vi "Get top coincs to check and grafts.vi"(11 "Coincidences":T1[](array[typedef])) -> (0 "Coincidences to check":T1[](array[typedef]), 1 "Found safe graft spot?":bool, 2 "Coincidences to graft":T1[](array[typedef]))   [LabVIEW 2016]
uses:
  Typedefs/Coincidence.ctl
  Global Variables/Global Resolution.vi
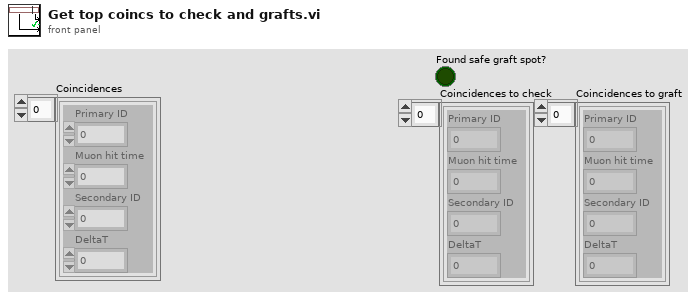
[diagram p1: front panel]
types:
  T1 = typedef "Coincidence.ctl" = cluster{"Primary ID":i8, "Muon hit time":u64, "Secondary ID":i8, "DeltaT":i32}
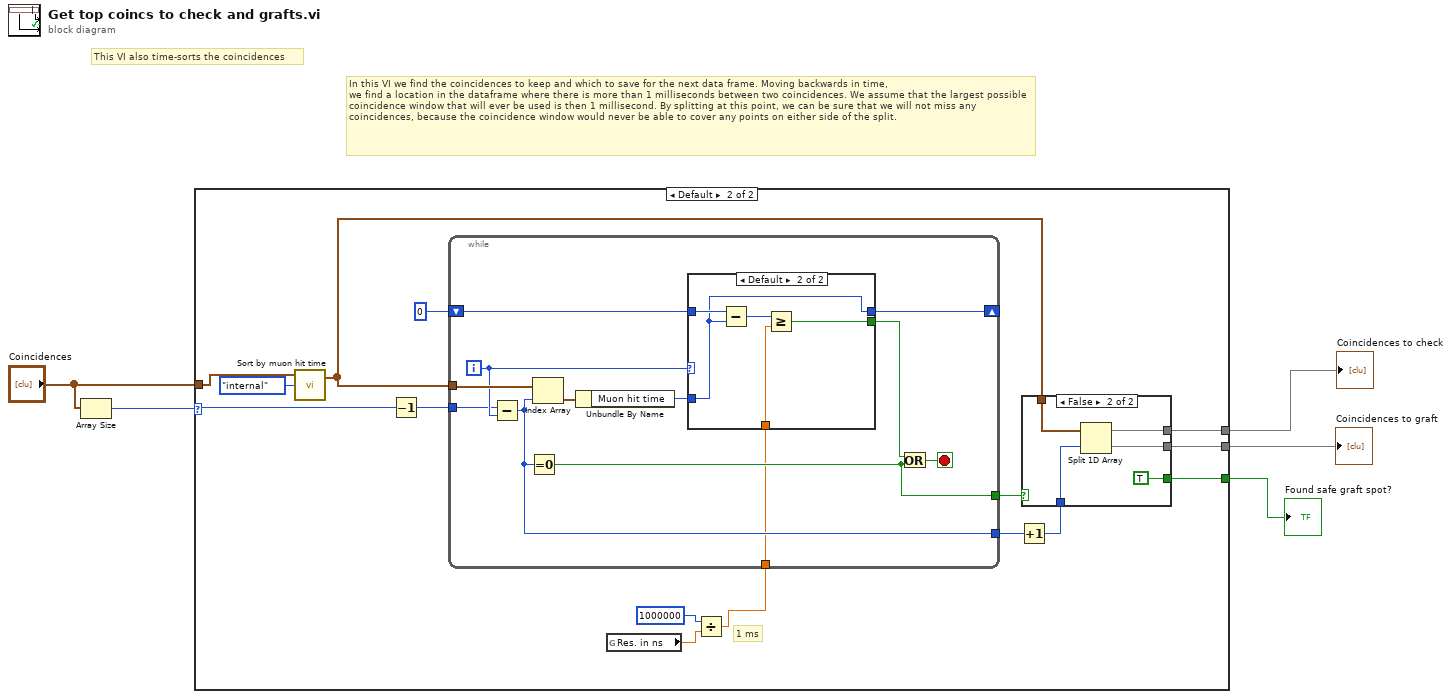
[diagram p0: block diagram]
diagram:
  # "This VI also time-sorts the coincidences"
  # "In this VI we find the coincidences to keep and which to save for the next data frame. Moving backwards in time,\nwe find a location in the dataframe where there is more than 1 milliseconds between two coincidences. We assume that the largest possible coincidence window that will ever be used is then 1 millisecond. By splitting at this point, we can be sure that we will not miss any coincidences, because the coincidence window would never be able to cover any points on either side of the split."
  n1 = Array Size(array="Coincidences") -> (size(s)=w2:i32)
  n2 = case shown="Default" w2 {
    selector: w2 -> [_ w14]
    tunnel: [_ w18] -> w5
    tunnel: [_ w17] -> w4
    tunnel: "Coincidences" -> [_ w8]
    tunnel: [_ w9] -> w1
    frame 0 {
    }
    frame Default {
      # "1 ms"
      n3 = call "Sort by muon hit time.vi"("Type"=enum16{"internal", "saving"}."internal", "Top Coincs internal"=w8) -> ("Coincidences internal"=w6:T1[])  [unwired: 1 in, 1 out]
      n4 = Decrement(x=w14) -> (x-1=w15:i32)
      n5 = global read "Global Resolution.vi" "Res. in ns"() -> (w11:ext)
      n6 = Divide(x=i64 1000000 ("y"), y=w11) -> (x/y=w10:ext)
      n7 = while {
        tunnel: w6 -> [w38]
        tunnel: [w36] -> w19
        shift-right: [w33] -> _
        shift-left: i64 0 ("Muon hit time") -> [w32]
        tunnel: w15 -> [w29]
        tunnel: [w28] -> w13
        tunnel: w10 -> [w27]
        i -> [w34]
        stop <- w31 stop-if-true
        n8 = Subtract(x=w29, y=w34) -> (x-y=w36:i32)
        n9 = Equal To 0?(x=w36) -> (x = 0?=w28:bool)
        n10 = Index Array(array=w38, index=w36) -> (element=w37:T1)
        n11 = Unbundle By Name(w37) -> ("Muon hit time"=w35:u64)
        n12 = case shown="Default" w34 {
          tunnel: w35 -> [w39 w42]
          tunnel: [w39 w42] -> w33
          tunnel: w32 -> [_ w44]
          tunnel: [_ w41] -> w30
          tunnel: w27 -> [_ w40]
          frame 0 {
          }
          frame Default {
            n13 = Subtract(x=w44, y=w42) -> (x-y=w43:u64)
            n14 = Greater Or Equal?(x=w43, y=w40) -> (x >= y?=w41:bool)
          }
        }
        n15 = Or(x=w30, y=w28) -> (x .or. y?=w31:bool)
      }
      n16 = Increment(x=w19) -> (x+1=w20:i32)
      n17 = case shown="False" w13 {
        tunnel: w20 -> [_ w26]
        tunnel: [_ w25] -> w18
        tunnel: [w21 w24] -> w17
        tunnel: w6 -> [w21 w23]
        tunnel: [_ TRUE] -> w9
        frame True {
        }
        frame False {
          n18 = Split 1D Array(array=w23, index=w26) -> (first subarray=w25:T1[], second subarray=w24:T1[])
        }
      }
    }
  }
  "Coincidences to check" <- w5
  "Coincidences to graft" <- w4
  "Found safe graft spot?" <- w1
